vi "10_ПростейшийВПс_Formula Node.vi"() -> ()   [LabVIEW 2016]
panel:
  out "Y":dbl
  in  "X":dbl
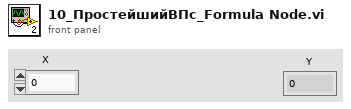
[diagram p1: front panel]
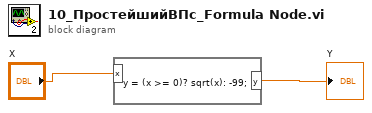
[diagram p0: block diagram]
diagram:
  n1 = formula code="y = (x >= 0)? sqrt(x): -99;"("x"="X") -> ("y"=→"Y":dbl)
